vi "Set Brightness.vi"(8 "error in":errorcluster, 11 "DMK33UP2000 in":refnum<class "DMK33UP2000.lvclass">) -> (0 "error out":errorcluster, 2 "Supported?":bool, 3 "DMK33UP2000 out":refnum<class "DMK33UP2000.lvclass">)   [LabVIEW 2018, in "DMK33UP2000.lvlib" / "DMK33UP2000.lvclass"]
uses:
  DMK33UP2000.lvclass
  builds/Camera.lvlibp/Camera.lvclass
  <resource>/objmgr/imaqdx.rc
  C:/Users/Ron.Dexter.LUMINARTECH/Desktop/builds/Camera.lvlibp/Camera.lvclass
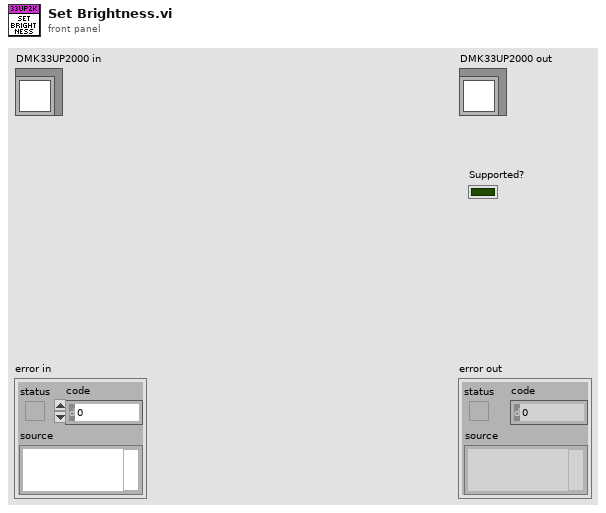
[diagram p1: front panel]
types:
  T1 = typedef "Camera.lvlibp/IMAQdx.ctl" = refnum<k21>
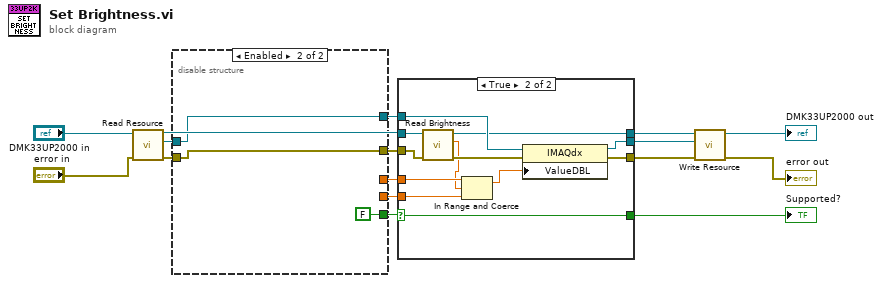
[diagram p0: block diagram]
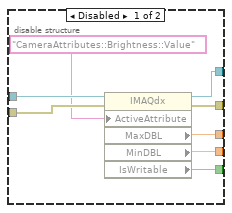
[diagram p2: hidden frame]
diagram:
  n1 = call "Read Resource.vi"("error in (no error)"="error in", "Camera in"="DMK33UP2000 in") -> ("error out"=w7:errorcluster, "IMAQdx Session"=w6:T1, "Camera out"=w11:refnum<class "DMK33UP2000.lvclass">)  [unwired: 7 in]
  n2 = disable-structure shown="Enabled" {
    disable-tunnel: [w24 _] -> w16
    disable-tunnel: [w23 _] -> w15
    disable-tunnel: [w22 w26] -> w13
    disable-tunnel: [w21 w27] -> w9
    disable-tunnel: [w20 FALSE ("IsWritable")] -> w8
    disable-tunnel: w7 -> [w19 w26]
    disable-tunnel: w6 -> [w18 w27]
    frame Disabled {
      n3 = property class="IMAQdx"(reference=w18, error in=w19, "ActiveAttribute"="CameraAttributes::Brightness::Value") -> (reference out=w21:T1, error out=w22:errorcluster, "MaxDBL"=w23:dbl, "MinDBL"=w24:dbl, "IsWritable"=w20:bool)
    }
    frame Enabled {
    }
  }
  n4 = case shown="True" w8 {
    selector: w8 -> [w29 w43]
    tunnel: [w29 w43] -> w1
    tunnel: w9 -> [w30 w42]
    tunnel: [w30 w41] -> w10
    tunnel: w11 -> [w31 w40]
    tunnel: [w31 w38] -> w12
    tunnel: w13 -> [w28 w37]
    tunnel: [w28 w36] -> w14
    tunnel: w15 -> [_ w35]
    tunnel: w16 -> [_ w34]
    frame False {
    }
    frame True {
      n5 = call "Read Brightness.vi"("error in (no error)"=w37, "Camera in"=w40) -> ("error out"=w39:errorcluster, "Brightness"=w32:dbl, "Camera out"=w38:refnum<class "DMK33UP2000.lvclass">)  [unwired: 7 in]
      n6 = In Range and Coerce(upper limit=w35, x=w32, lower limit=w34) -> (coerced(x)=w33:dbl)  [unwired: 1 out]
      n7 = property class="IMAQdx"(reference=w42, error in=w39, "ValueDBL"=w33) -> (reference out=w41:T1, error out=w36:errorcluster)
    }
  }
  "Supported?" <- w1
  n8 = call "Write Resource.vi"("error in (no error)"=w14, "IMAQdx Session"=w10, "Camera in"=w12) -> ("error out"=→"error out":errorcluster, "Camera out"=→"DMK33UP2000 out":refnum<class "DMK33UP2000.lvclass">)  [unwired: 7 in]
